vi "Update History Data (Boolean).vi"(7 "reset?":bool, 10 "new data":bool, 11 "History Data In":bool[](array[boolean])) -> (3 "History Data Out":bool[](array[boolean]))   [LabVIEW 2017, in "SoundVib_Resampling.lvlib"]
uses:
  <vilib>/addons/Sound and Vibration/Order Analysis/Resample Order Tracking/SoundVib_Resampling.lvlib
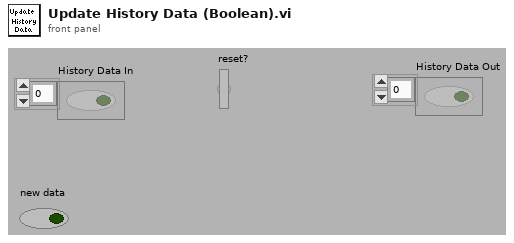
[diagram p1: front panel]
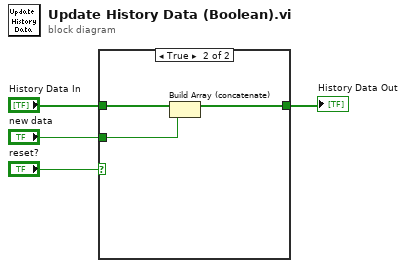
[diagram p0: block diagram]
diagram:
  n1 = case shown="True" "reset?" {
    tunnel: "History Data In" -> [w5 w8]
    tunnel: "new data" -> [_ w7]
    tunnel: [w5 w6] -> w2
    frame False {
    }
    frame True {
      n2 = Build Array (concatenate)(w8, w7) -> (w6:bool[])
    }
  }
  "History Data Out" <- w2
